vi "Save Image backup.vi"(8 "Data":dbl[][](array[numeric]), 10 "Process Index":i32, 11 "Current File Num":i32) -> ()   [LabVIEW 2013]
uses:
  <vilib>/Utility/file.llb/Write To Spreadsheet File (I64).vi
panel:
  out "Path Prefix":string
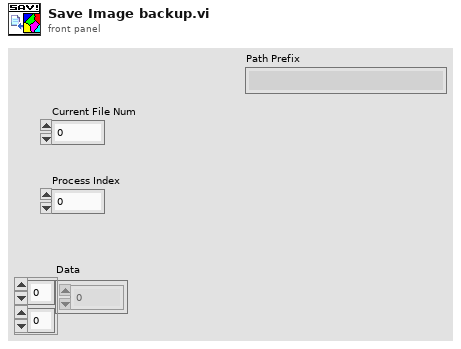
[diagram p1: front panel]
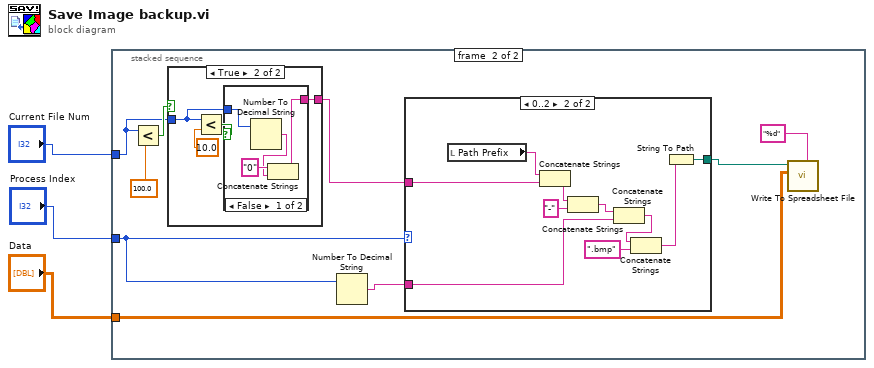
[diagram p0: block diagram]
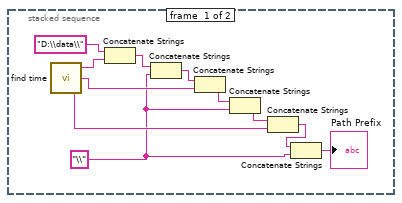
[diagram p2: hidden frame]
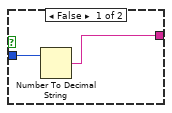
[diagram p3: hidden frame]
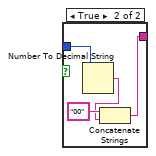
[diagram p4: hidden frame]
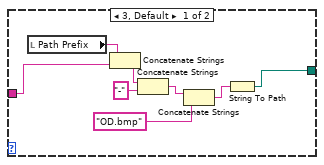
[diagram p5: hidden frame]
diagram:
  n1 = stacked-sequence {
    tunnel: "Current File Num" -> [_ w17]
    tunnel: "Process Index" -> [_ w21]
    tunnel: "Data" -> [_ w22]
    frame #0 {
      w5 = "\\" ("字符串")
      n2 = call "find time.vi"() -> ("day"=w7:string, "month"=w10:string, "year"=w13:string)  [unwired: 3 in]
      n3 = Concatenate Strings("D:\\data\\", w13) -> (w12:string)
      n4 = Concatenate Strings(w12, w5) -> (w11:string)
      n5 = Concatenate Strings(w11, w10) -> (w9:string)
      n6 = Concatenate Strings(w9, w5) -> (w8:string)
      n7 = Concatenate Strings(w8, w7) -> (w6:string)
      n8 = Concatenate Strings(w6, w5) -> (→"Path Prefix":string)
    }
    frame #1 {
      n9 = Less?(x=w17, y=100.0) -> (x < y?=w18:bool)
      n10 = case shown="True" w18 {
        tunnel: w17 -> [w25 w27]
        tunnel: [w24 w26] -> w16
        frame False {
          n11 = Number To Decimal String(number=w25) -> (decimal integer string=w24:string)  [unwired: 1 in]
        }
        frame True {
          n12 = Less?(x=w27, y=10.0) -> (x < y?=w28:bool)
          n13 = case shown="False" w28 {
            tunnel: w27 -> [w32 w37]
            tunnel: [w30 w34] -> w26
            frame False {
              n14 = Number To Decimal String(number=w32) -> (decimal integer string=w31:string)  [unwired: 1 in]
              n15 = Concatenate Strings("0" ("字符串"), w31) -> (w30:string)
            }
            frame True {
              n16 = Number To Decimal String(number=w37) -> (decimal integer string=w35:string)  [unwired: 1 in]
              n17 = Concatenate Strings("00" ("字符串"), w35) -> (w34:string)
            }
          }
        }
      }
      n18 = Number To Decimal String(number=w21) -> (decimal integer string=w20:string)  [unwired: 1 in]
      n19 = case shown="0..2" w21 {
        tunnel: [w38 w54] -> w23
        tunnel: w16 -> [w41 w53]
        tunnel: w20 -> [_ w49]
        frame 3, Default {
          n20 = local read "Path Prefix"() -> (w42:string)
          n21 = Concatenate Strings(w42, w41) -> (w45:string)
          n22 = Concatenate Strings(w45, "-" ("字符串")) -> (w43:string)
          n23 = Concatenate Strings(w43, "OD.bmp" ("字符串")) -> (w39:string)
          n24 = String To Path(string=w39) -> (path=w38:path)
        }
        frame 0..2 {
          n25 = local read "Path Prefix"() -> (w55:string)
          n26 = Concatenate Strings(w55, w53) -> (w52:string)
          n27 = Concatenate Strings(w52, "-" ("字符串")) -> (w50:string)
          n28 = Concatenate Strings(w50, w49) -> (w47:string)
          n29 = Concatenate Strings(w47, ".bmp" ("字符串")) -> (w48:string)
          n30 = String To Path(string=w48) -> (path=w54:path)
        }
      }
      n31 = call-poly <vilib>:"Write To Spreadsheet File.vi"("format (%d)"="%d", "2D data"=w22, "file path (dialog if empty)"=w23) -> ()  [unwired: 5 in, 1 out]
    }
  }
